vi "FileMan Open File.vi"(0 "error in (no error)":errorcluster, 1 "run minimized (F)":bool, 2 "default directory (empty path)":path, 5 "path to file (empty path)":path, 6 "command line parameters (\"\")":string) -> (3 "error out":errorcluster)   [LabVIEW 2011]
doc: "This VI will open a file whose extension is associated with an application, as available in Windows' File Manager, just as if you double-clicked on the file in File Manager. For example, files with the .wri extension are usually associated with the Windows application Write (write.exe). A file with the extension .wri will then be opened by Microsoft Write.\n\nAttempting to open files whose extensions are not associated with an application in the File Manager will result in an error."
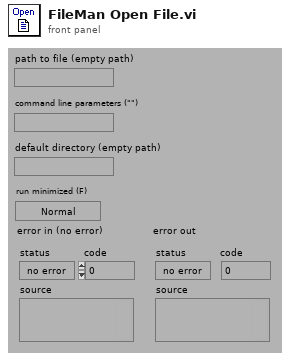
[diagram p1: front panel]
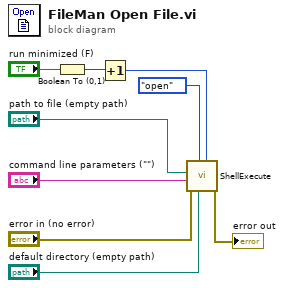
[diagram p0: block diagram]
diagram:
  n1 = Boolean To (0,1)(Boolean="run minimized (F)") -> (0, 1=w1:i16)
  n2 = Increment(x=w1) -> (x+1=w3:i16)
  n3 = call "ShellExecute.vi"("show"=w3, "default directory"="default directory (empty path)", "operation (open)"=enum16{"open", "print"}."open", "error in (no error)"="error in (no error)", "command line parameters"="command line parameters (\"\")", "path to file"="path to file (empty path)") -> ("error out"=→"error out":errorcluster)  [unwired: 1 in, 4 out]
